vi "Global-test-int.vi"() -> ()   [LabVIEW 2020, in "Sgraph_lib_V1.lvlib"]
uses:
  Builds/Sgraph_lib_V1.lvlib
panel:
  in  "H-shift-test":i32
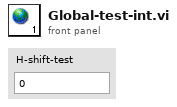
[diagram p1: front panel]
diagram:
